vi "Add Glyph to VIs.vi"() -> ()   [LabVIEW 2012]
doc: "Requests the user to select one or more VIs, to then add the <b>Glyph</b> to each VI's icon."
panel:
  in  "Glyph":path
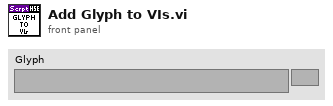
[diagram p1: front panel]
types:
  T1 = typedef "imagedata.ctl" = cluster{"image type":i32, "image depth":i32, "image":u8[], "mask":u8[], "colors":u32[], "Rectangle":cluster{"left":i16, "top":i16, "right":i16, "bottom":i16}}
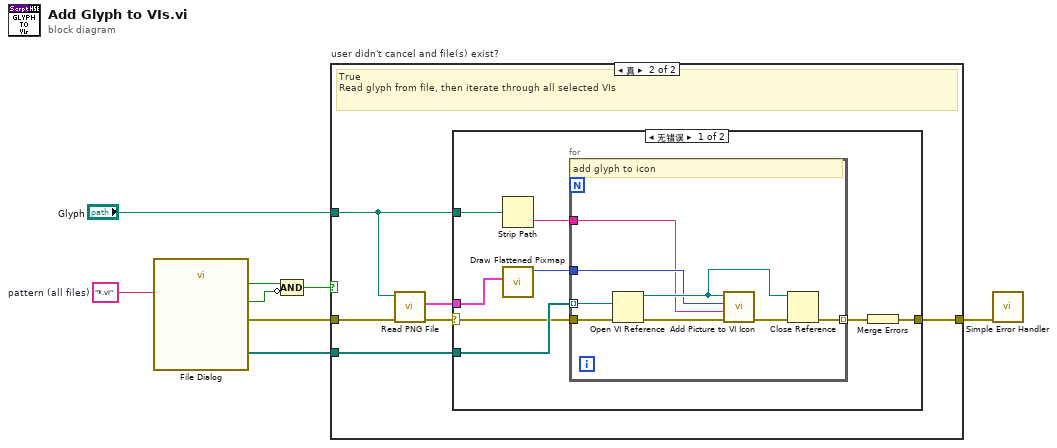
[diagram p0: block diagram]
diagram:
  w5 = "*.vi"  # pattern (all files)
  n1 = call "File Dialog"("pattern (all files)"=w5) -> ("selected paths"=w6:path[], "exists"=w3:bool, "cancelled"=w2:bool, "error out"=w8:errorcluster)  [unwired: 11 in]
  n2 = Compound Arithmetic op=AND(w3, invert w2) -> (w1:bool)
  n3 = case "user didn't cancel and file(s) exist?" shown="真" w1 {
    tunnel: w8 -> [w9 w15]
    tunnel: "Glyph" -> [_ w14]
    tunnel: w6 -> [_ w12]
    tunnel: [w9 w11] -> w4
    frame False {
      # "False\nDo nothing."
    }
    frame True {
      # "True\nRead glyph from file, then iterate through all selected VIs"
      n4 = call <vilib>:"Read PNG File.vi"("error in (no error)"=w15, "path to PNG file"=w14) -> ("error out"=w10:errorcluster, "image data"=w13:T1)  [unwired: 7 in, 1 out]
      n5 = case shown="无错误" w10 {
        selector: w10 -> [w16 w32]
        tunnel: w14 -> [w23 _]
        tunnel: w13 -> [w22 _]
        tunnel: w12 -> [w19 _]
        tunnel: [w17 w32] -> w11
        frame No Error {
          n6 = Strip Path(path=w23) -> (name=w20:string)  [unwired: 1 out]
          n7 = call <vilib>:"Draw Flattened Pixmap.vi"("image data"=w22) -> ("new picture"=w21:picture)  [unwired: 8 in]
          n8 = for {
            tunnel: w16 -> [w26]
            tunnel: w21 -> [w29]
            tunnel: w20 -> [w28]
            tunnel: w19 -> [w27] mode=indexing
            tunnel: [w24] -> w18 mode=indexing
            # "add glyph to icon"
            n9 = Open VI Reference(vi path=w27, error in (no error)=w26) -> (vi reference=w31:refnum<vi>, error out=w30:errorcluster)  [unwired: 4 in]
            n10 = call "Add Picture to VI Icon.vi"("error in (no error)"=w30, "Layer Name"=w28, "Picture"=w29, "VI Reference"=w31) -> ("error out"=w25:errorcluster)  [unwired: 7 in]
            n11 = Close Reference(reference=w31, error in (no error)=w25) -> (error out=w24:errorcluster)
          }
          n12 = Merge Errors(w18) -> (w17:errorcluster)
        }
        frame Error {
        }
      }
    }
  }
  n13 = call <vilib>:"Simple Error Handler.vi"("error in (no error)"=w4) -> ()  [unwired: 4 in, 5 out]
